vi "UpdateComm.vi"(8 "error in (no error)":errorcluster, 11 "Sync Box in":refnum<class "Sync Box.lvclass">) -> (0 "error out":errorcluster, 3 "Sync Box out":refnum<class "Sync Box.lvclass">)   [LabVIEW 2018, in "Sync Box.lvclass"]
uses:
  Sync Box.lvclass
  Sync Box.lvclass/Sync Box.ctl
  Device/Device.lvclass/Device.ctl
  Trigger/Trigger.lvclass
  C:/Users/observer/Desktop/Sparc4GUI/SPARC4_GUI/Device/Device.lvclass
  Server/Server.lvclass
  StateMachine/State Machine.lvclass
  Device/Device.lvclass
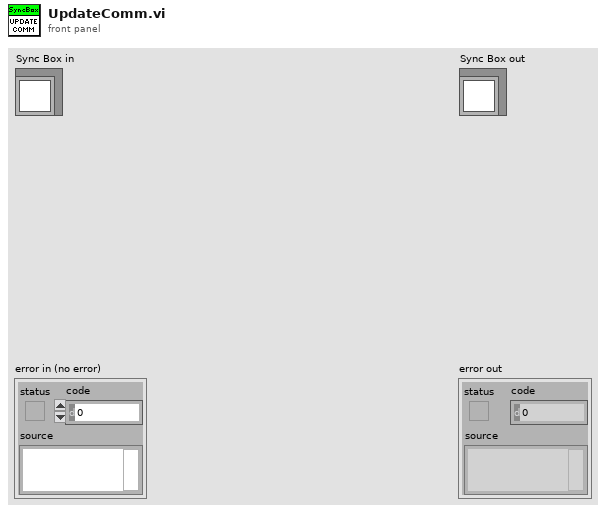
[diagram p1: front panel]
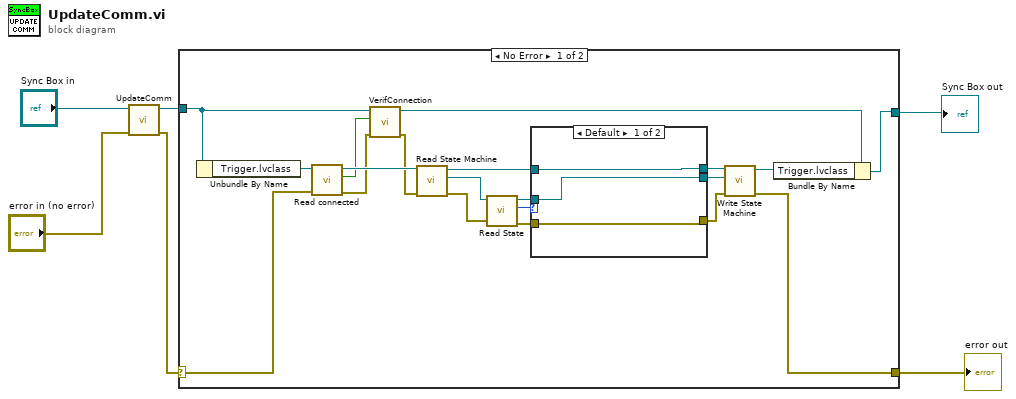
[diagram p0: block diagram]
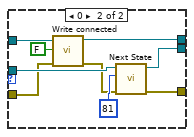
[diagram p2: hidden frame]
diagram:
  n1 = call-parent "UpdateComm.vi"("error in (no error)"="error in (no error)", "Server in"="Sync Box in") -> ("error out"=w1:errorcluster, "Server out"=w4:refnum<class "Sync Box.lvclass">)  [unwired: 8 in]
  n2 = case shown="No Error" w1 {
    selector: w1 -> [w23 w40]
    tunnel: [w7 w40] -> w2
    tunnel: [w8 w39] -> w3
    tunnel: w4 -> [w13 w39]
    frame No Error {
      n3 = Unbundle By Name(w13) -> ("Trigger.lvclass"=w24:refnum<class "Trigger.lvclass">)
      n4 = call "Read connected.vi"("error in (no error)"=w23, "Device in"=w24) -> ("error out"=w11:errorcluster, "connected"=w12:bool, "Device out"=w22:refnum<class "Trigger.lvclass">)  [unwired: 7 in]
      n5 = call-dynamic "VerifConnection.vi"("error in (no error)"=w11, "device connected in"=w12, "Server in"=w13) -> ("error out"=w10:errorcluster, "Server out"=w9:refnum<class "Sync Box.lvclass">)  [unwired: 7 in]
      n6 = call-dynamic "Read State Machine.vi"("error in (no error)"=w10, "Device in"=w22) -> ("error out"=w18:errorcluster, "State Machine.lvclass"=w26:refnum<class "State Machine.lvclass">, "Device out"=w21:refnum<class "Trigger.lvclass">)  [unwired: 7 in]
      n7 = call-dynamic "Read State.vi"("error in (no error)"=w18, "State Machine in"=w26) -> ("error out"=w17:errorcluster, "State"=w25:i32, "State Machine out"=w20:refnum<class "State Machine.lvclass">)  [unwired: 7 in]
      n8 = case shown="Default" w25 {
        tunnel: w21 -> [w29 w37]
        tunnel: w20 -> [w28 w36]
        tunnel: [w28 w34] -> w19
        tunnel: w17 -> [w27 w32]
        tunnel: [w27 w31] -> w16
        tunnel: [w29 w30] -> w15
        frame Default {
        }
        frame 0 {
          n9 = call "Write connected.vi"("error in (no error)"=w32, "connected"=FALSE, "Device in"=w37) -> ("error out"=w33:errorcluster, "Device out"=w30:refnum<class "Trigger.lvclass">)  [unwired: 7 in]
          n10 = call "Next State.vi"("error in (no error)"=w33, "New_State"=81, "State Machine in"=w36) -> ("error out"=w31:errorcluster, "State Machine out"=w34:refnum<class "State Machine.lvclass">)  [unwired: 7 in]
        }
      }
      n11 = call-dynamic "Write State Machine.vi"("error in (no error)"=w16, "State Machine.lvclass"=w19, "Device in"=w15) -> ("error out"=w7:errorcluster, "Device out"=w14:refnum<class "Trigger.lvclass">)  [unwired: 7 in]
      n12 = Bundle By Name(cluster=w9, "Trigger.lvclass"=w14) -> (w8:refnum<class "Sync Box.lvclass">)
    }
    frame Error {
    }
  }
  "error out" <- w2
  "Sync Box out" <- w3
